vi "cast u-64-64 to u64.vi"(11 "fixedpoint_i":fxp<+,64,64>) -> (3 "aifxp":u64)   [LabVIEW 2019, in "fixedpoint-cast.lvlib"]
uses:
  fixedpoint-cast.lvlib
  <vilib>/rvi/IPIntegrationNode/IPINode_Typedef/niFpgaIPINodeSupportedFamilies.ctl
  <vilib>/rvi/IPIntegrationNode/IPINode_Utilities/niFpgaIPINodeSimCore.vi
  <vilib>/rvi/IPIntegrationNode/IPINode_Xnode/niFpgaIPINode.xnode
  fixedpoint_vhdl/src/cast_u_dash_64_dash_64_to_u64SimFiles/xsim.dir/fixedpoint_to_u64/xsimk3948EAE62C9749CEA36883D0D40AEC2A.dll
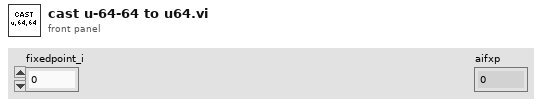
[diagram p1: front panel]
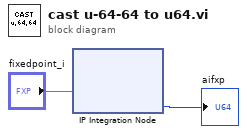
[diagram p0: block diagram]
diagram:
  n1 = xnode "IP Integration Node"("fixedpoint_i"="fixedpoint_i") -> ("u64_o"=→"aifxp":u64)
